vi "svc_Convert Array of Peaks to XY Format.vi"(4 "peaks":cluster{"frequency [Hz]":dbl, "amplitude":dbl}[](array[cluster]) {"amplitude" format="%.2f"; "frequency [Hz]" format="%.2f"}) -> (1 "peaks":cluster{"X":dbl[], "Y":dbl[]} {"Y" format="%.2f"; "X" format="%.2f"})   [LabVIEW 2017]
doc: "Converts an array of peaks of the form [{x y}] to an XY output of the form {[X] [Y]}. Peaks equal to {0 0} are not included in the output."
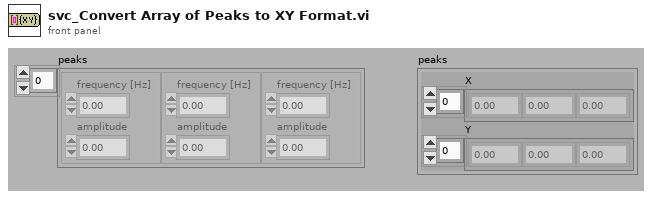
[diagram p1: front panel]
types:
  T1 = cluster{"frequencies [Hz]":dbl[], "values":dbl[]}
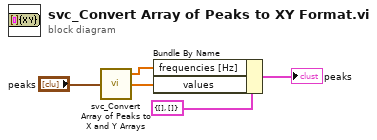
[diagram p0: block diagram]
diagram:
  n1 = call <vilib>:"svc_Convert Array of Peaks to X and Y Arrays.vi"("peaks"="peaks") -> ("Y"=w1:dbl[], "X"=w2:dbl[])  [unwired: 3 in]
  n2 = Bundle By Name(cluster=T1 {"frequencies [Hz]"=[], "values"=[]} ("lower limit 2"), "frequencies [Hz]"=w2, "values"=w1) -> (→"peaks":T1)
